vi "Generate Bezier Trajectory.vi"(6 "Overrides":T3(array[cluster]), 7 "dynamic?":bool, 8 "Conditions":T5, 9 "Limits":T4={"Velocity (fps)"=6.0, "Accel (fps^2)"=15.0, "Jerk (fps^3)"=150.0, "StoopidFast (fps)"=6.0} {"StoopidFast (fps)" min=0.0; "Jerk (fps^3)" min=0.0 step=1.0; "Accel (fps^2)" min=0.0; "Velocity (fps)" min=0.0}, 10 "percision":sgl, 11 "WayPoints":T6) -> (0 "Time & Dist":cluster{"Time (s)":dbl, "Distance (ft)":dbl}, 1 "Valid":bool, 2 "Updated Waypoints":cluster{"x":dbl, "y":dbl, "th":dbl}[](array[cluster]), 3 "Trajectory Data":T1)   [LabVIEW 2019]
uses:
  Types/Waypoints.ctl
  Types/Limits.ctl
  Types/Trajectory Data.ctl
  Types/Segment Type.ctl
panel:
  out "x-y":u32
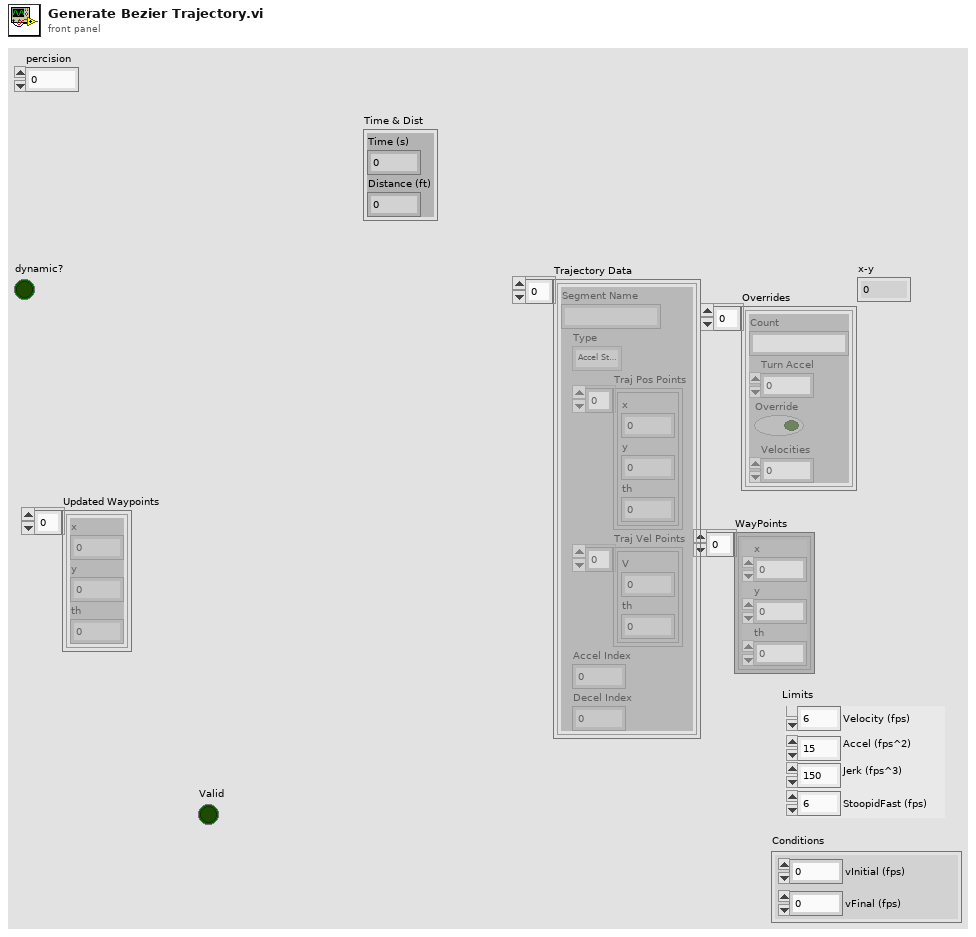
[diagram p1: front panel]
types:
  T1 = typedef "Trajectory Data.ctl" = cluster{"Segment Name":string, "Type":T2, "Traj Pos Points":cluster{"x":dbl, "y":dbl, "th":dbl}[], "Traj Vel Points":cluster{"V":dbl, "th":dbl}[], "Accel Index":i32, "Decel Index":i32}[]
  T2 = typedef "Segment Type.ctl" = enum16{"Accel Straight", "Const Straight", "Blend", "Circle", "Bezier"}
  T3 = cluster{"Count":string, "Turn Accel":dbl, "Override":bool, "Velocities":dbl}[]
  T4 = typedef "Limits.ctl" = cluster{"Velocity (fps)":dbl, "Accel (fps^2)":dbl, "Jerk (fps^3)":dbl, "StoopidFast (fps)":dbl}
  T5 = cluster{"vInitial (fps)":dbl, "vFinal (fps)":dbl}
  T6 = typedef "Waypoints.ctl" = cluster{"x":sgl, "y":sgl, "th":sgl}[]
  T7 = cluster{"Velocity (fps)":dbl, "Accel (fps^2)":dbl, "Jerk (fps^3)":dbl}
  T8 = typedef "Bezier Curve.ctl" = cluster{"x":sgl, "y":sgl}[]
  T9 = cluster{"Segment Name":string, "Type":T2, "Traj Pos Points":cluster{"x":dbl, "y":dbl, "th":dbl}[], "Traj Vel Points":cluster{"V":dbl, "th":dbl}[], "Accel Index":i32, "Decel Index":i32}
  T10 = cluster{"Segment Name":string, "Type":T2, "Traj Pos Points":cluster{"x":dbl, "y":dbl, "th":dbl}[], "Traj Vel Points":cluster{"V":dbl, "th":dbl}[], "Accel Index":i32, "Decel Index":i32}[]
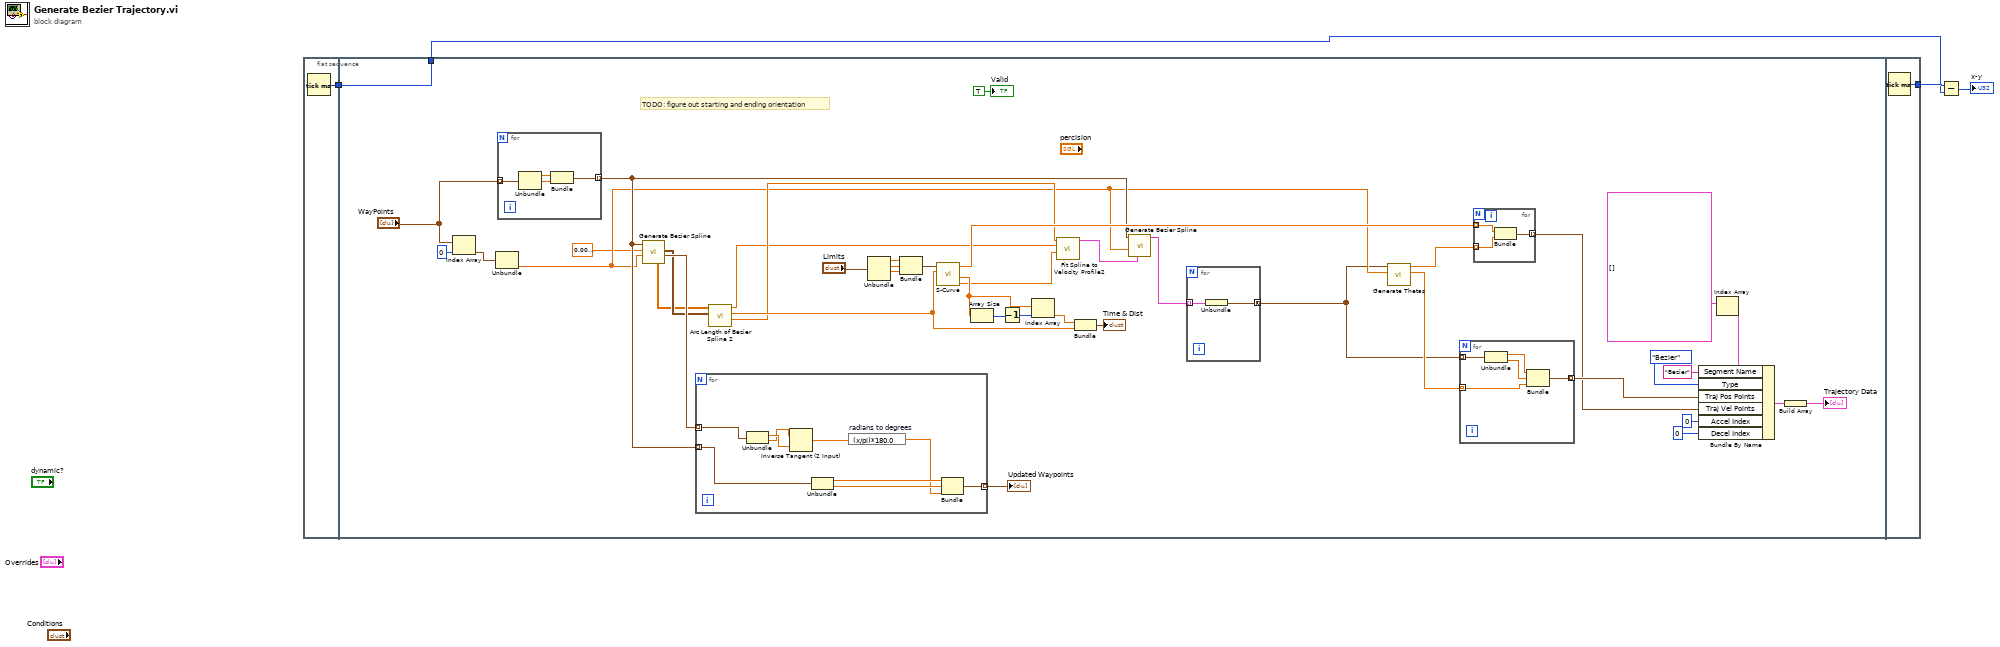
[diagram p0: block diagram]
diagram:
  n1 = flat-sequence {
    tunnel: [w5] -> w3
    tunnel: [w23] -> w2
    tunnel: w3 -> [w23]
    tunnel: [w71] -> w4
    frame #0 {
      n2 = Tick Count (ms)() -> (millisecond timer value=w5:u32)
    }
    frame #1 {
      # "TODO: figure out starting and ending orientation"
      n3 = Index Array(array="WayPoints", index=0) -> (element=w46:cluster{"x":sgl, "y":sgl, "th":sgl})
      n4 = Unbundle(w46) -> ("th"=w11:sgl)  [unwired: 2 out]
      n5 = for {
        tunnel: "WayPoints" -> [w62] mode=indexing
        tunnel: [w59] -> w13 mode=indexing
        n6 = Unbundle(w62) -> ("x"=w61:sgl, "y"=w60:sgl)  [unwired: 1 out]
        n7 = Bundle("x"=w61, "y"=w60) -> (w59:cluster{"x":sgl, "y":sgl})  [unwired: 1 in]
      }
      n8 = call "Generate Bezier Spline.vi"("starting orientation"=w11, "percision"=sgl 0.01, "waypts"=w13) -> ("Tangents"=w40:cluster{sgl, sgl}[], "ctrl pts"=w19:cluster{sgl, sgl}[][], "position out"=w8:sgl[][])  [unwired: 4 in, 2 out]
      n9 = for {
        tunnel: w13 -> [w58] mode=indexing
        tunnel: w40 -> [w50] mode=indexing
        tunnel: [w55] -> w21 mode=indexing
        n10 = Unbundle(w50) -> (w53:sgl, w52:sgl)
        n11 = Inverse Tangent (2 Input)(1:w53, 2:w52) -> (0:w51:sgl)
        n12 = Unbundle(w58) -> ("x"=w57:sgl, "y"=w56:sgl)
        n13 = expression code="(x/pi)*180.0" "radians to degrees"(w51) -> (w54:sgl)
        n14 = Bundle("x"=w57, "y"=w56, w54) -> (w55:cluster{"x":sgl, "y":sgl, sgl})  [unwired: 1 in]
      }
      "Updated Waypoints" <- w21
      n15 = call "Arc Length of Bezier Spline 2.vi"("ctrl pts"=w19, "position"=w8) -> ("t"=w16:sgl[], "l total"=w18:dbl, "l"=w15:dbl[])  [unwired: 6 in, 1 out]
      n16 = Unbundle("Limits") -> ("Velocity (fps)"=w44:dbl, "Accel (fps^2)"=w43:dbl, "Jerk (fps^3)"=w42:dbl)  [unwired: 1 out]
      n17 = Bundle("Velocity (fps)"=w44, "Accel (fps^2)"=w43, "Jerk (fps^3)"=w42) -> (w41:T7)  [unwired: 1 in]
      n18 = call "S-Curve.vi"("goal"=w18, "Limits"=w41) -> ("X"=w12:dbl[], "T"=w14:dbl[], "V"=w34:dbl[])  [unwired: 6 in, 1 out]
      n19 = Array Size(array=w14) -> (size(s)=w39:i32)
      n20 = Decrement(x=w39) -> (x-1=w38:i32)
      n21 = Index Array(array=w14, index=w38) -> (element=w37:dbl)
      n22 = call "Fit Spline to Velocity Profile2.vi"("vel positions"=w12, "s(t)"=w15, "t flat"=w16) -> ("y unflat"=w10:cluster{dbl[]}[])  [unwired: 8 in]
      n23 = Bundle(w37, "l total"=w18) -> (→"Time & Dist":cluster{dbl, "l total":dbl})  [unwired: 1 in]
      n24 = call "Generate Bezier Spline.vi"("positions"=w10, "starting orientation"=w11, "waypts"=w13) -> ("bezier spline"=w7:cluster{"curve ":T8}[])  [unwired: 4 in, 4 out]
      n25 = for {
        tunnel: w7 -> [w49] mode=indexing
        tunnel: [w48] -> w6 mode=concatenating
        n26 = Unbundle(w49) -> ("curve"=w48:T8)
      }
      n27 = call "Generate Thetas.vi"("starting angle"=w11, "spline flat"=w6) -> ("theta"=w20:sgl[], "dtheta"=w22:sgl[])  [unwired: 8 in]
      n28 = for {
        tunnel: w6 -> [w67] mode=indexing
        tunnel: [w64] -> w29 mode=indexing
        tunnel: w20 -> [w63] mode=indexing
        n29 = Unbundle(w67) -> ("x"=w66:sgl, "y"=w65:sgl)
        n30 = Bundle("x"=w66, "y"=w65, w63) -> (w64:cluster{"x":sgl, "y":sgl, sgl})  [unwired: 1 in]
      }
      n31 = for {
        tunnel: w22 -> [w69] mode=indexing
        tunnel: w34 -> [w70] mode=indexing
        tunnel: [w68] -> w28 mode=indexing
        n32 = Bundle(w70, w69) -> (w68:cluster{dbl, sgl})  [unwired: 1 in]
      }
      n33 = Index Array(array=T1 [] ("Trajectory Data")) -> (element=w32:T9)  [unwired: 1 in]
      n34 = Bundle By Name(cluster=w32, "Segment Name"="Bezier", "Type"=Segment_Type."Bezier", "Traj Pos Points"=w29, "Traj Vel Points"=w28, "Accel Index"=0, "Decel Index"=0) -> (w25:T9)
      n35 = Build Array(w25) -> (→"Trajectory Data":T10)
      "Valid" <- TRUE ("Valid")
    }
    frame #2 {
      n36 = Tick Count (ms)() -> (millisecond timer value=w71:u32)
    }
  }
  n37 = Subtract(x=w4, y=w2) -> (x-y=→"x-y":u32)
